vi "fft per channel.vi"(8 "sample in":T1, 9 "valid":bool, 10 "FIFO FFT CPX IMAG In":refnum<k21>, 11 "FIFO FFT CPX REAL In":refnum<k21>) -> (2 "sample out":T2, 3 "m_axis_data_tvalid":bool)   [LabVIEW 2020]
uses:
  <vilib>/rvi/IPIntegrationNode/IPINode_Typedef/niFpgaIPINodeSupportedFamilies.ctl
  <vilib>/rvi/IPIntegrationNode/IPINode_Utilities/niFpgaIPINodeSimCore.vi
  <vilib>/rvi/DataTransferAndStorage/Container/Common/niFpgaContainerExecOnDevCompGetState.vi
  <vilib>/rvi/Emulation/niFpgaEmulationIsFPGAContextNoSignature.vi
  <vilib>/rvi/Emulation/niFpgaSctlEmulationGetInTimedLoop.vi
  <vilib>/rvi/errors/niFpgaSetErrorForExecOnDevCompSimple.vi
  <vilib>/rvi/eio/common/nirviEmuReportErrorAndStop.vi
  <vilib>/rvi/DataTransferAndStorage/Container/Common/niFpgaContainerGetUniqueNameForEmu.vi
  <vilib>/rvi/FIFO/Fifo_Resource/nirvififoEmulationSetSize.vi
  <vilib>/rvi/FIFO/Fifo_Resource/nirviFifoEmulationQueueMgr.vi
  <instcachedir>/0/nirviFifoEmulationQueueMgr_E5CAEC123FF24DC58D834DCA3CDAA9B5.lvgen/nirviFifoEmulationQueueMgr_E5CAEC123FF24DC58D834DCA3CDAA9B5_010.vi
  <vilib>/rvi/FIFO/Fifo_Resource/nirvififoEmulationDetermineInputValidOut.vi
  <vilib>/rvi/FIFO/Fifo_Resource/nirvififoEmulationCreateLock.vi
  <vilib>/rvi/Emulation/niFpgaProcessEmulError.vi
  <vilib>/rvi/FIFO/Fifo_Resource/nirvififoEmulationObtainLock.vi
  <vilib>/rvi/FIFO/Fifo_Resource/nirvififoEmulationReleaseLock.vi
  <vilib>/rvi/occurrence/nirviWaitOnOccurrenceBase.vi
  <vilib>/rvi/errors/nirviReportUnexpectedCaseInternalError.vi
  <vilib>/rvi/errors/nirviReportUnexpectedCaseInternalError (U32).vi
  <vilib>/Utility/error.llb/Clear Errors.vi
  <vilib>/rvi/interface/RandomDataEmulation/niFpgaRandomDataHandleErrors.vi
  <vilib>/rvi/XilinxIP/XIPIN_XNode/niFpgaXIPIN.xnode
  fft per channel/Fast Fourier Transform/xsim.dir/Fast_Fourier_Transform_695370033AFB4392836E8ED390166882/xsimk_695370033AFB4392836E8ED390166882.dll
  <vilib>/rvi/IPIntegrationNode/IPINode_Xnode/niFpgaIPINode.xnode
  <vilib>/rvi/FXPMathLib/FxpInterpret/XNode/nifxpmath_Interpret.xnode
  <vilib>/rvi/DataTransferAndStorage/Container/XNode/niFpgaContainer.xnode
  <vilib>/rvi/FIFO/Fifo_Resource/niFpgaFifoEmulationRefIn.vi
  <instrlib>/_niInstr/Basic Elements/v1/FPGA/niInstr Basic Elements v1 FPGA.lvlib
types:
  T1 = cluster{"Real":fxp<+/-,16,3>, "Imag":fxp<+/-,16,3>}
  T2 = cluster{"Real":fxp<+/-,25,4>, "Imag":fxp<+/-,25,4>}
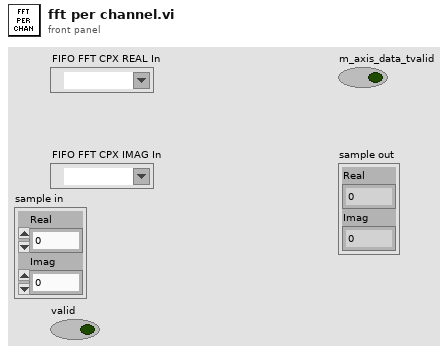
[diagram p1: front panel]
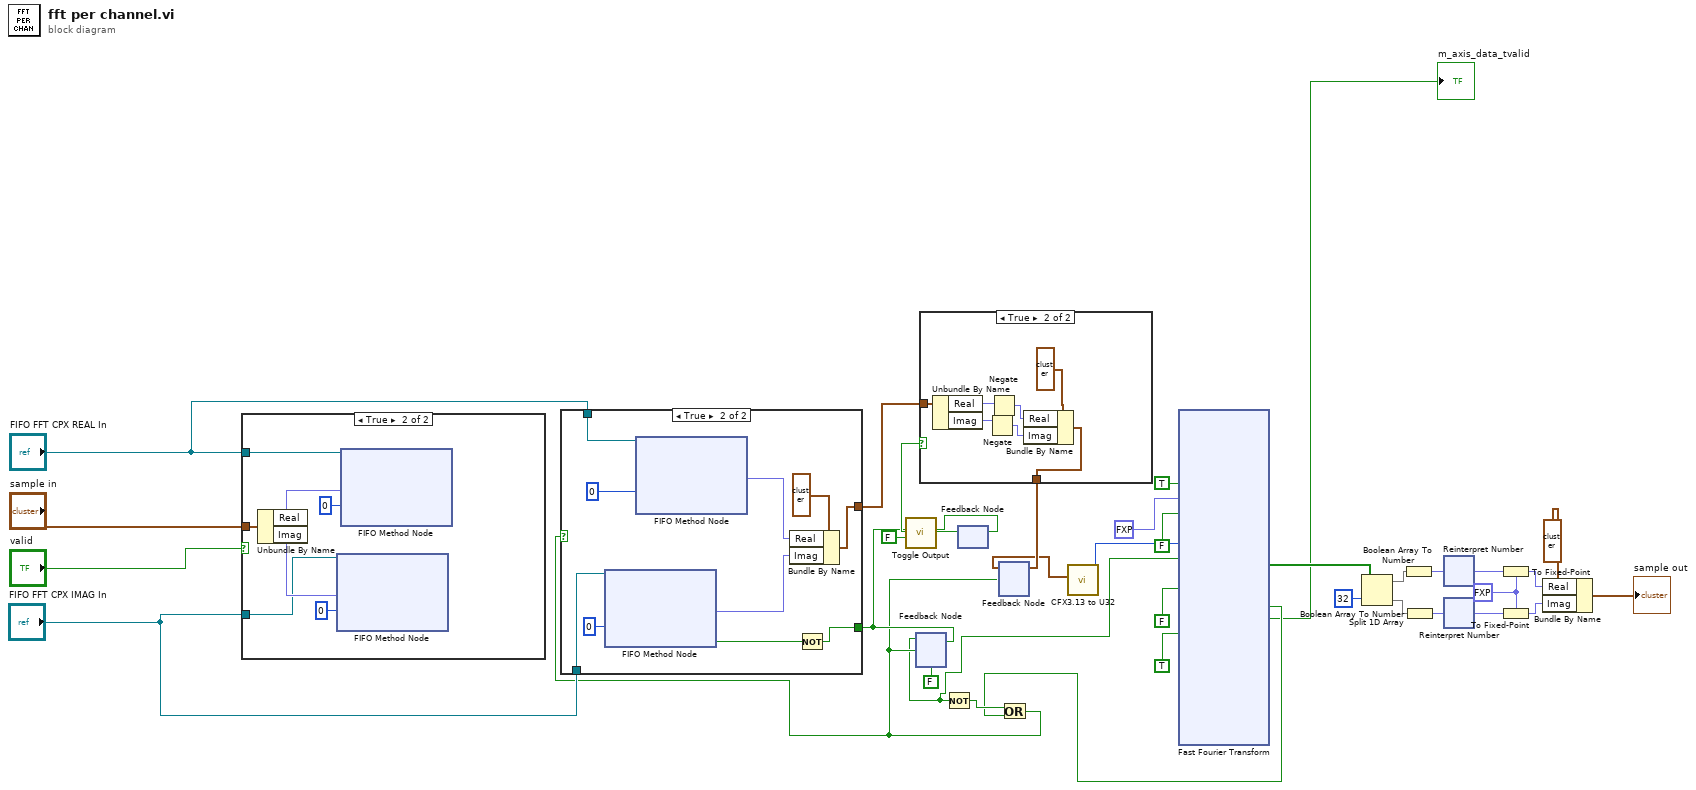
[diagram p0: block diagram]
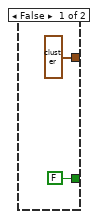
[diagram p3: hidden frame]
diagram:
  w28 = fxp<+/-,25,4> 0.0 ("fixed-point type")
  n1 = case shown="True" "valid" {
    tunnel: "sample in" -> [_ w41]
    tunnel: "FIFO FFT CPX REAL In" -> [_ w38]
    tunnel: "FIFO FFT CPX IMAG In" -> [_ w37]
    frame False {
    }
    frame True {
      n2 = Unbundle By Name(w41) -> ("Real"=w40:fxp<+/-,16,3>, "Imag"=w39:fxp<+/-,16,3>)
      n3 = xnode ("FIFO Method Node")("Element"=w39, "Timeout"=0, "FIFO In"=w37) -> ()  [unwired: 2 out]
      n4 = xnode ("FIFO Method Node")("Element"=w40, "Timeout"=0, "FIFO In"=w38) -> ()  [unwired: 2 out]
    }
  }
  n5 = feedback #1(FALSE) -> (w15:bool)
  n6 = Not(x=w15) -> (.not. x?=w13:bool)
  n7 = feedback #2() -> (w22:bool)  [unwired: 1 in]
  n8 = feedback #3() -> (w17:T1)  [unwired: 1 in]
  n9 = call "CFX3.13 to U32.vi"("Data in"=w17) -> ("Data out"=w2:u32)  [unwired: 10 in]
  n10 = xnode ("Fast Fourier Transform")("aclken"=TRUE, "s_axis_config_tdata"=fxp<+,8,8> 0.0, "s_axis_config_tvalid"=FALSE, "s_axis_data_tdata"=w2, "s_axis_data_tvalid"=w15, "s_axis_data_tlast"=FALSE, "m_axis_data_tready"=TRUE) -> ("s_axis_data_tready"=w11:bool, "m_axis_data_tdata"=w9:bool[], "m_axis_data_tvalid"=→"m_axis_data_tvalid":bool)  [unwired: 8 out]
  n11 = Or(x=w13, y=w11) -> (x .or. y?=w16:bool)
  n12 = case shown="True" w16 {
    tunnel: [FALSE w49] -> w18
    tunnel: [T1 {"Real"=0.0, "Imag"=0.0} ("sample in") w48] -> w21
    tunnel: "FIFO FFT CPX REAL In" -> [_ w47]
    tunnel: "FIFO FFT CPX IMAG In" -> [_ w46]
    frame False {
    }
    frame True {
      n13 = xnode ("FIFO Method Node")("Timeout"=0, "FIFO In"=w46) -> ("Element"=w51:fxp<+/-,16,3>, "Timed Out?"=w50:bool)  [unwired: 1 out]
      n14 = xnode ("FIFO Method Node")("Timeout"=0, "FIFO In"=w47) -> ("Element"=w52:fxp<+/-,16,3>)  [unwired: 2 out]
      n15 = Bundle By Name(cluster=T1 {"Real"=0.0, "Imag"=0.0} ("sample in"), "Real"=w52, "Imag"=w51) -> (w48:T1)
      n16 = Not(x=w50) -> (.not. x?=w49:bool)
    }
  }
  n17 = call <instrlib>:"Toggle Output.vi"("clear"=FALSE, "toggle"=w18) -> ("output"=w20:bool)  [unwired: 9 in]
  n18 = feedback-in #1(w18, w16) -> ()
  n19 = case shown="True" w22 {
    tunnel: w21 -> [w56 w63]
    tunnel: [w56 w57] -> w23
    frame False {
    }
    frame True {
      n20 = Unbundle By Name(w63) -> ("Real"=w62:fxp<+/-,16,3>, "Imag"=w61:fxp<+/-,16,3>)
      n21 = Negate(x=w61) -> (-x=w58:fxp<+/-,16,3>)
      n22 = Negate(x=w62) -> (-x=w59:fxp<+/-,16,3>)
      n23 = Bundle By Name(cluster=T1 {"Real"=0.0, "Imag"=0.0} ("sample in"), "Real"=w59, "Imag"=w58) -> (w57:T1)
    }
  }
  n24 = feedback-in #2(w20) -> ()
  n25 = feedback-in #3(w23, w16) -> ()
  n26 = Split 1D Array(array=w9, index=32) -> (first subarray=w24:bool[], second subarray=w25:bool[])
  n27 = Boolean Array To Number(Boolean array=w24) -> (number=w26:fxp<+/-,32,19>)
  n28 = Boolean Array To Number(Boolean array=w25) -> (number=w27:fxp<+/-,32,19>)
  n29 = xnode "Reinterpret Number"("x"=w26) -> ("y"=w29:fxp<+/-,32,11>)
  n30 = xnode "Reinterpret Number"("x"=w27) -> ("y"=w30:fxp<+/-,32,11>)
  n31 = To Fixed-Point(fixed-point type=w28, number=w29) -> (fixed-point=w33:fxp<+/-,25,4>)
  n32 = To Fixed-Point(fixed-point type=w28, number=w30) -> (fixed-point=w34:fxp<+/-,25,4>)
  n33 = Bundle By Name(cluster=T2 {"Real"=0.0, "Imag"=0.0} ("sample in"), "Real"=w33, "Imag"=w34) -> (→"sample out":T2)
